vi "四人表决逻辑电路.vi"() -> ()   [LabVIEW 2018]
panel:
  in  "结束":bool
  out "布尔":bool
  in  "D":bool
  in  "C":bool
  in  "B":bool
  in  "A":bool
  # "74HC151：八选一数据选择器\n74HC00：与非门"
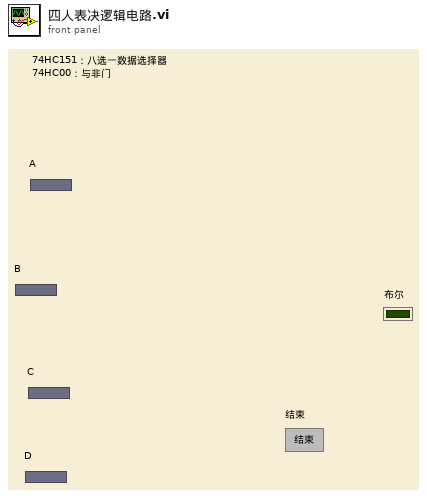
[diagram p1: front panel]
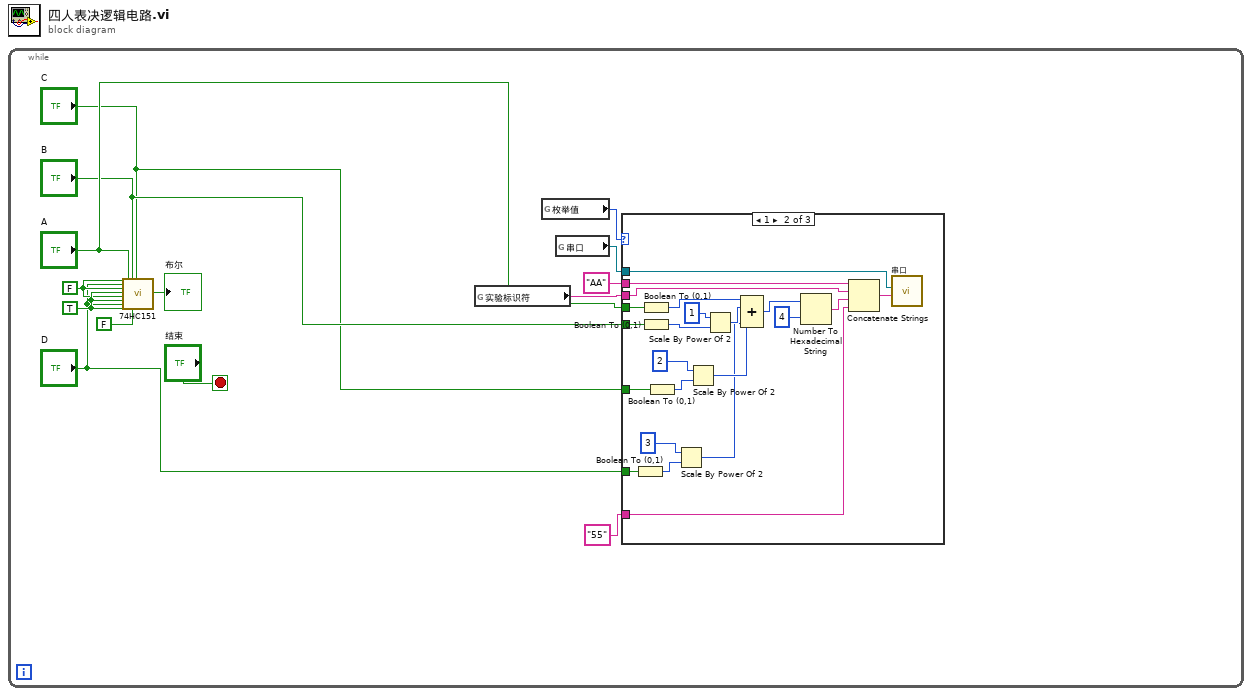
[diagram p0: block diagram]
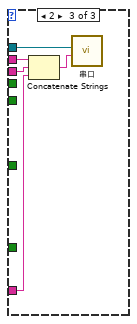
[diagram p3: hidden frame]
diagram:
  n1 = while {
    stop <- "结束" stop-if-true
    w11 = FALSE
    w12 = TRUE
    n2 = call "74HC151.vi"("D 0"=w11, "D 1"="D", "D 2"=w11, "D 3"=w12, "D 4"=w11, "D 5"=w12, "D 6"="D", "D 7"=w12, "A0"="A", "A1"="B", "EN"=FALSE, "A2"="C") -> ("布尔"=→"布尔":bool)  [unwired: 15 in]
    n3 = global read "全局变量.vi" "实验标识符"() -> (w7:string)
    n4 = global read "全局变量.vi" "枚举值"() -> (w9:i8)
    n5 = global read "全局变量.vi" "串口"() -> (w8:refnum<visa-resource-name>)
    n6 = case shown="1" w9 {
      tunnel: "B" -> [_ w31 _]
      tunnel: "A" -> [_ w30 _]
      tunnel: w8 -> [_ w29 w39]
      tunnel: w7 -> [_ w28 w40]
      tunnel: "55" -> [_ w27 w37]
      tunnel: "AA" -> [_ w26 w38]
      tunnel: "C" -> [_ w20 _]
      tunnel: "D" -> [_ w15 _]
      frame 0, Default {
      }
      frame 1 {
        n7 = Boolean To (0,1)(Boolean=w15) -> (0, 1=w18:i16)
        n8 = Boolean To (0,1)(Boolean=w30) -> (0, 1=w35:i16)
        n9 = Boolean To (0,1)(Boolean=w31) -> (0, 1=w33:i16)
        n10 = Boolean To (0,1)(Boolean=w20) -> (0, 1=w21:i16)
        n11 = Scale By Power Of 2(n=3, x=w18) -> (x*2^n=w16:i16)
        n12 = Scale By Power Of 2(n=2, x=w21) -> (x*2^n=w22:i16)
        n13 = Scale By Power Of 2(n=1, x=w33) -> (x*2^n=w34:i16)
        n14 = Compound Arithmetic op=ADD ("复合运算")(w35, w34, w22, w16) -> (w25:i16)
        n15 = Number To Hexadecimal String(1:4, 2:w25) -> (0:w23:string)
        n16 = Concatenate Strings(w26, w28, w23, w27) -> (w36:string)
        n17 = call "串口.vi"("字符串"=w36, "VISA resource name"=w29) -> ()  [unwired: 10 in]
      }
      frame 2 {
        n18 = Concatenate Strings(w38, w40, w37) -> (w41:string)
        n19 = call "串口.vi"("字符串"=w41, "VISA resource name"=w39) -> ()  [unwired: 10 in]
      }
    }
  }
